vi "U8Array2ZplString.vi"(1 "in Array":u8[](array[numeric])=array[76000 elements]) -> (0 "字符串":string)   [LabVIEW 2018]
panel:
  out "最大值":u8
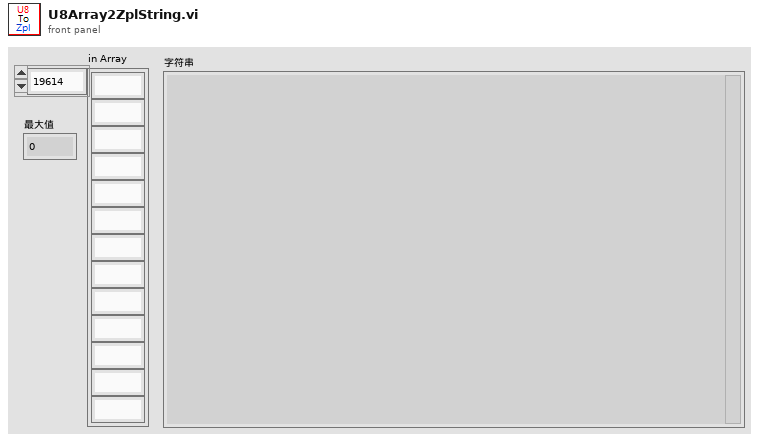
[diagram p1: front panel]
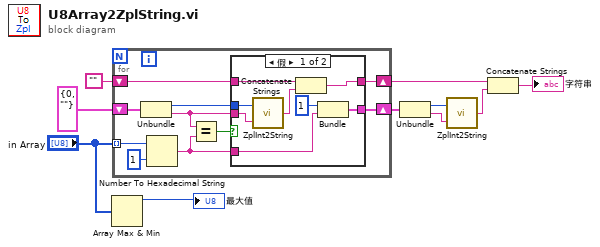
[diagram p0: block diagram]
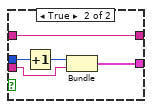
[diagram p2: hidden frame]
diagram:
  n1 = Array Max & Min(array="in Array") -> (max value=→"最大值":u8)  [unwired: 3 out]
  n2 = for {
    shift-right: [w14] -> w8
    shift-left: cluster{i32, string} {0, ""} -> [w17]
    tunnel: "in Array" -> [w19] mode=indexing
    shift-right: [w12] -> w4
    shift-left: "" -> [w11]
    n3 = Unbundle(w17) -> (w15:i32, w16:string)
    n4 = Number To Hexadecimal String(1:i16 1 ("宽度(-)"), 2:w19) -> (0:w13:string)
    n5 = Equal?(x=w16, y=w13) -> (x = y?=w18:bool)
    n6 = case shown="假" w18 {
      tunnel: w16 -> [w27 w31]
      tunnel: w15 -> [w28 w33]
      tunnel: [w24 w30] -> w14
      tunnel: w13 -> [w25 _]
      tunnel: [w22 w29] -> w12
      tunnel: w11 -> [w21 w29]
      frame False {
        n7 = call "ZplInt2String.vi"("字符"=w27, "Int"=w28) -> ("outString"=w23:string)
        n8 = Concatenate Strings(w21, w23) -> (w22:string)
        n9 = Bundle(1, w25) -> (w24:cluster{i32, string})  [unwired: 1 in]
      }
      frame True {
        n10 = Increment(x=w33) -> (x+1=w32:i32)
        n11 = Bundle(w32, w31) -> (w30:cluster{i32, string})  [unwired: 1 in]
      }
    }
  }
  n12 = Unbundle(w8) -> (w7:i32, w6:string)
  n13 = call "ZplInt2String.vi"("字符"=w6, "Int"=w7) -> ("outString"=w5:string)
  n14 = Concatenate Strings(w4, w5) -> (→"字符串":string)
